vi "Main.vi"() -> ()   [LabVIEW 2019]
doc: "This template is for the Queued Message Handler design pattern.\n\nThe Event Handling Loop generates messages based on user interface actions.\n\nThe Message Handling Loop processes messages generated by the Event Handling Loop, or by other messages. The messages are string values, so new messages can be added easily to the Message Cases case structure in the Message Handling Loop. Each message cluster can also provide an optional value for Message Data, which is a variant that can be converted to whatever message-specific data is required."
uses:
  Firebase.lvclass
  controls/UI Data.ctl
  support/Message Queue/Enqueue Message (Single).vi
  <vilib>/Platform/browser.llb/Open URL in Default Browser (string).vi
  <vilib>/Utility/error.llb/Error Cluster From Error Code.vi
  <vilib>/ErrorRing/Error Ring.xnode
  support/Message Queue/Message Queue.lvlib
  support/User Event - Stop/User Event - Stop.lvlib
panel:
  in  "OPERARIO":string
  in  "Firebase in":refnum<class "Firebase.lvclass">
  out "Firebase out":refnum<class "Firebase.lvclass">
  in  "HUMEDAD ACTUAL":dbl
  in  "TEMPERATURA ACTUAL":dbl
  in  "PH ACTUAL":dbl
  in  "VER BASE DE DATOS":bool
  in  "ACTUALIZAR HUMEDAD":bool
  in  "ACTUALIZAR TEMPERATURA":bool
  in  "ACTUALIZAR PH":bool
  in  "Exit":bool
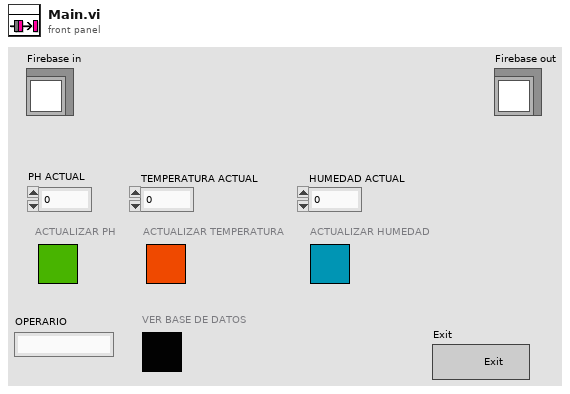
[diagram p1: front panel]
types:
  T1 = typedef "UI Data.ctl" = cluster{"Boolean <Replace Me>":bool, "String <Replace Me>":string, "Numeric <Replace Me>":dbl, "Do Something Ref":refnum<vi>, "Do Something Else Ref":refnum<vi>, "Data Display Ref":refnum<vi>, "Exit Button Ref":refnum<vi>, "OPERARIO":string, "url":string}
  T2 = typedef "Message Queue.lvlib/All Message Queues.ctl" = cluster{"UI":refnum<queue>}
  T3 = cluster{"Fecha":timestamp, "PH":dbl, "Humeda":dbl, "Temperatura":dbl, "Operario":string}
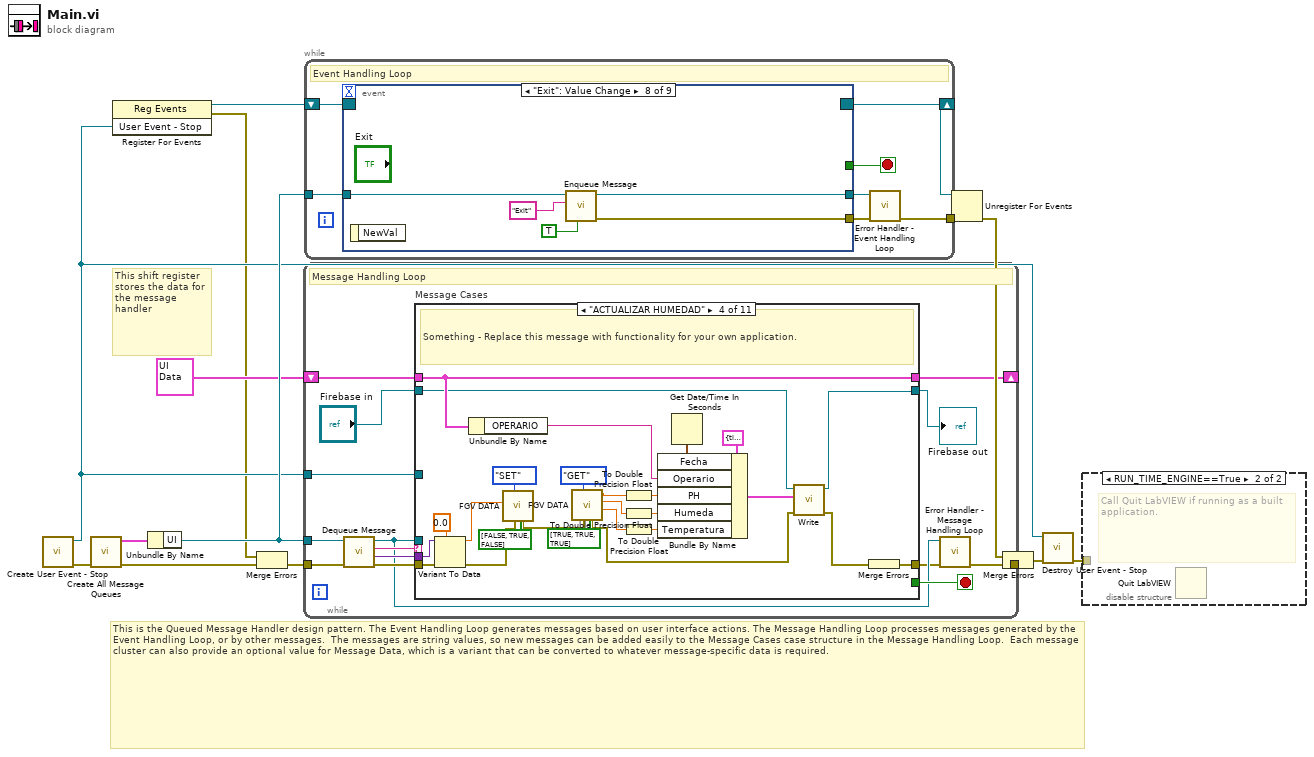
[diagram p0: block diagram]
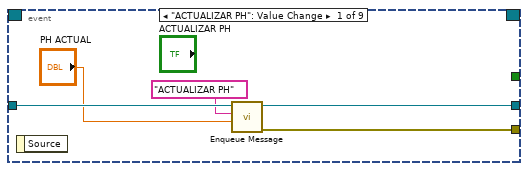
[diagram p3: hidden frame]
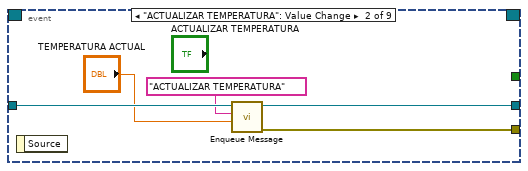
[diagram p4: hidden frame]
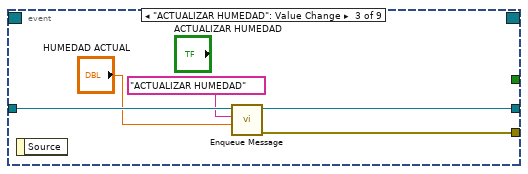
[diagram p5: hidden frame]
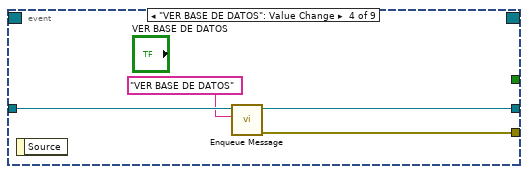
[diagram p6: hidden frame]
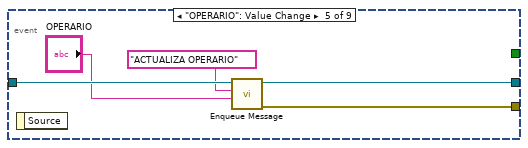
[diagram p7: hidden frame]
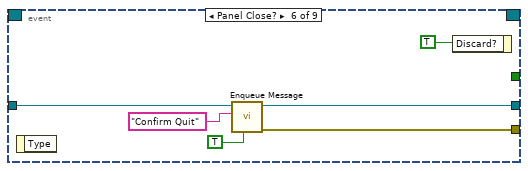
[diagram p8: hidden frame]
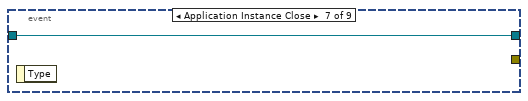
[diagram p9: hidden frame]
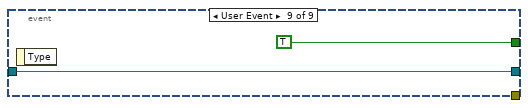
[diagram p10: hidden frame]
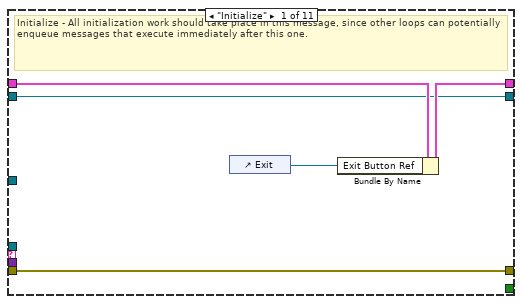
[diagram p11: hidden frame]
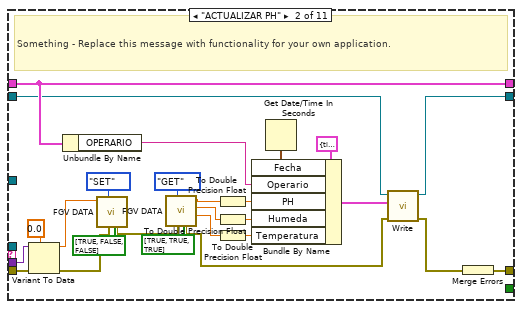
[diagram p12: hidden frame]
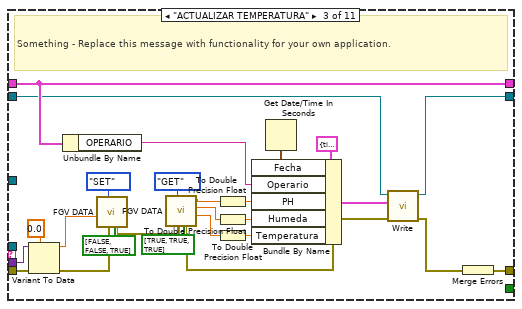
[diagram p13: hidden frame]
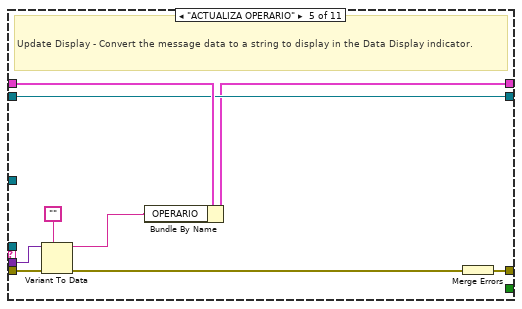
[diagram p14: hidden frame]
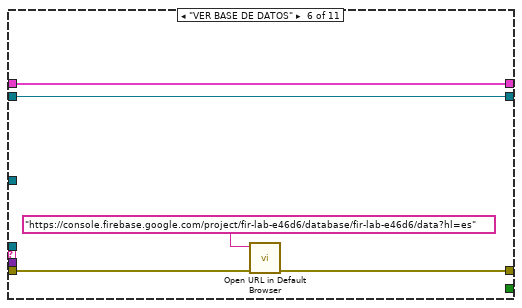
[diagram p15: hidden frame]
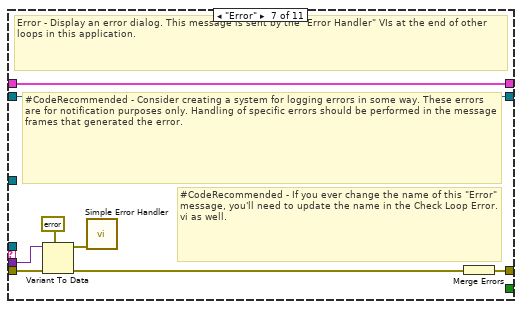
[diagram p16: hidden frame]
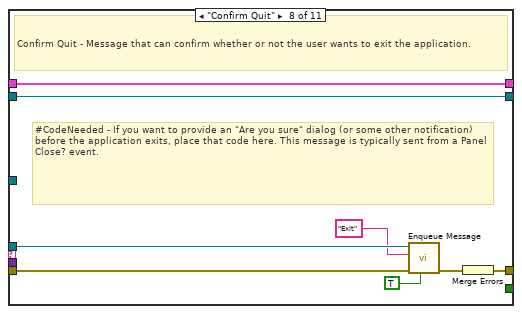
[diagram p17: hidden frame]
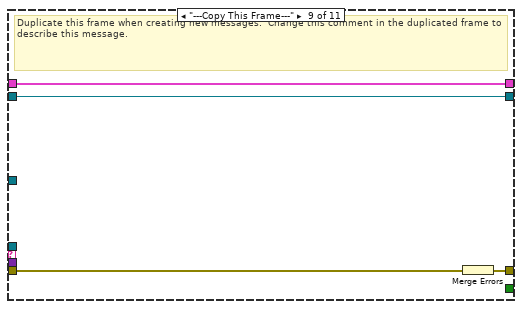
[diagram p18: hidden frame]
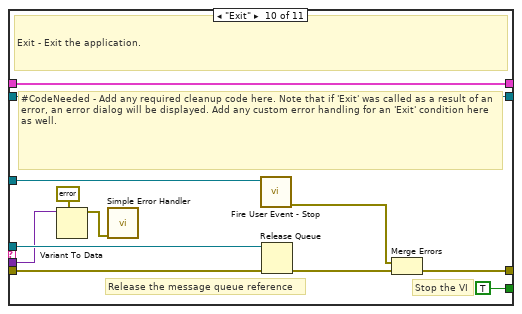
[diagram p19: hidden frame]
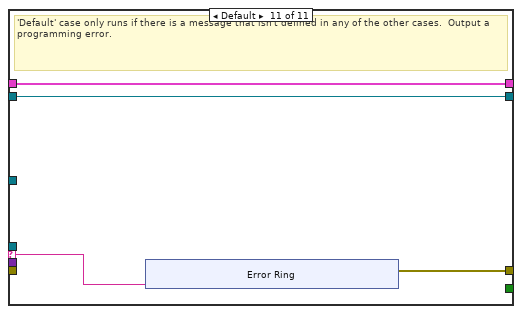
[diagram p20: hidden frame]
diagram:
  # "This is the Queued Message Handler design pattern. The Event Handling Loop generates messages based on user interface actions. The Message Handling Loop processes messages generated by the Event Handling Loop, or by other messages.  The messages are string values, so new messages can be added easily to the Message Cases case structure in the Message Handling Loop.  Each message cluster can also provide an optional value for Message Data, which is a variant that can be converted to whatever message-specific data is required."
  # "This shift register stores the data for the message handler"
  n1 = call "Create User Event - Stop.vi"() -> ("error out"=w11:errorcluster, "User Event - Stop"=w3:refnum<user-event>)  [unwired: 10 in]
  n2 = call "Create All Message Queues.vi"("error in (no error)"=w11) -> ("error out"=w15:errorcluster, "Message Queues out"=w14:T2)  [unwired: 9 in]
  n3 = register-events(w3) -> (reference out=w4:refnum<event-registration>, error out=w1:errorcluster)  [unwired: 2 in]
  n4 = Unbundle By Name(w14) -> ("UI"=w12:refnum<queue>)
  n5 = Merge Errors(w1, w15) -> (w2:errorcluster)
  n6 = while {
    tunnel: w12 -> [w21]
    shift-right: [w28] -> _
    shift-left: T1 {"Boolean <Replace Me>"=FALSE, "String <Replace Me>"="", "Numeric <Replace Me>"=0.0, "Do Something Ref"=refnum, "Do Something Else Ref"=refnum, "Data Display Ref"=refnum, "Exit Button Ref"=refnum, "OPERARIO"="", "url"=""} ("Data Cluster") -> [w29]
    tunnel: w3 -> [w26]
    tunnel: w2 -> [w25]
    tunnel: [w19] -> w13
    stop <- w27 stop-if-true
    # "Message Handling Loop"
    n7 = call "Dequeue Message.vi"("error in (no error)"=w25, "Message Queue"=w21) -> ("error out"=w24:errorcluster, "Message Data"=w22:variant, "Message"=w23:string, "dup Message Queue"=w20:refnum<queue>)  [unwired: 6 in]
    n8 = case "Message Cases" shown="\"ACTUALIZAR HUMEDAD\"" w23 {
      selector: w23 -> [_ _ _ _ _ _ _ _ _ _ w160]
      tunnel: w20 -> [_ _ _ _ _ _ _ w138 _ w158 _]
      tunnel: w24 -> [w34 w59 w85 w111 w119 w123 w134 w142 w146 w151 _]
      tunnel: [w34 w60 w86 w112 w120 w122 w128 w140 w144 w154 w161] -> w18
      tunnel: w29 -> [w33 w43 w71 w96 w121 w126 w133 w141 w145 w157 w162]
      tunnel: [w32 w43 w71 w96 w114 w126 w133 w141 w145 w157 w162] -> w28
      tunnel: [_ _ _ _ _ _ _ _ _ TRUE _] -> w27
      tunnel: w22 -> [_ w38 w66 w92 w118 _ w132 _ _ w148 _]
      tunnel: w26 -> [_ _ _ _ _ _ _ _ _ w153 _]
      tunnel: [w30 w40 w68 w90 w115 w125 w127 w135 w143 w147 w159] -> w17
      tunnel: "Firebase in" -> [w30 w41 w69 w94 w115 w125 w127 w135 w143 w147 w159]
      frame "Initialize" {
        # "Initialize - All initialization work should take place in this message, since other loops can potentially enqueue messages that execute immediately after this one."
        n9 = control-ref of="Exit"() -> (w31:refnum<vi>)
        n10 = Bundle By Name(cluster=w33, "Exit Button Ref"=w31) -> (w32:T1)
      }
      frame "ACTUALIZAR PH" {
        # "Something - Replace this message with functionality for your own application."
        n11 = Variant To Data(error in=w59, type=0.0, Variant=w38) -> (data=w56:dbl, error out=w37:errorcluster)
        n12 = Unbundle By Name(w43) -> ("OPERARIO"=w42:string)
        n13 = call "FGV DATA.vi"("error in (no error)"=w37, "Enum"=enum16{"SET", "GET"}."SET", "SET??"=bool[] [TRUE, FALSE, FALSE], "PH IN"=w56) -> ("error out"=w36:errorcluster)  [unwired: 4 in, 3 out]
        n14 = call "FGV DATA.vi"("error in (no error)"=w36, "Enum"=enum16{"SET", "GET"}."GET", "SET??"=bool[] [TRUE, TRUE, TRUE]) -> ("TEMPERATURA OUT"=w47:dbl, "HUMEDAD OUT"=w48:dbl, "PH OUT"=w49:dbl, "error out"=w35:errorcluster)  [unwired: 5 in]
        n15 = To Double Precision Float(number=w49) -> (double precision float=w50:dbl)
        n16 = To Double Precision Float(number=w48) -> (double precision float=w51:dbl)
        n17 = To Double Precision Float(number=w47) -> (double precision float=w52:dbl)
        n18 = Get Date/Time In Seconds() -> (seconds since 1Jan1904=w44:timestamp)
        n19 = Bundle By Name(cluster=T3 {"Fecha"=timestamp(0 s since 1904-01-01), "PH"=0.0, "Humeda"=0.0, "Temperatura"=0.0, "Operario"=""} ("dato"), "Fecha"=w44, "Operario"=w42, "PH"=w50, "Humeda"=w51, "Temperatura"=w52) -> (w45:T3)
        n20 = call "Write.vi"("error in (no error)"=w35, "dato"=w45, "Firebase in"=w41) -> ("error out"=w39:errorcluster, "Firebase out"=w40:refnum<class "Firebase.lvclass">)  [unwired: 6 in, 1 out]
        n21 = Merge Errors(w39) -> (w60:errorcluster)
      }
      frame "ACTUALIZAR TEMPERATURA" {
        # "Something - Replace this message with functionality for your own application."
        n22 = Variant To Data(error in=w85, type=0.0, Variant=w66) -> (data=w65:dbl, error out=w63:errorcluster)
        n23 = Unbundle By Name(w71) -> ("OPERARIO"=w70:string)
        n24 = call "FGV DATA.vi"("error in (no error)"=w63, "Enum"=enum16{"SET", "GET"}."SET", "SET??"=bool[] [FALSE, FALSE, TRUE], "TEMPERATURA IN"=w65) -> ("error out"=w62:errorcluster)  [unwired: 4 in, 3 out]
        n25 = call "FGV DATA.vi"("error in (no error)"=w62, "Enum"=enum16{"SET", "GET"}."GET", "SET??"=bool[] [TRUE, TRUE, TRUE]) -> ("TEMPERATURA OUT"=w75:dbl, "HUMEDAD OUT"=w76:dbl, "PH OUT"=w77:dbl, "error out"=w61:errorcluster)  [unwired: 5 in]
        n26 = To Double Precision Float(number=w77) -> (double precision float=w78:dbl)
        n27 = To Double Precision Float(number=w76) -> (double precision float=w79:dbl)
        n28 = To Double Precision Float(number=w75) -> (double precision float=w80:dbl)
        n29 = Get Date/Time In Seconds() -> (seconds since 1Jan1904=w72:timestamp)
        n30 = Bundle By Name(cluster=T3 {"Fecha"=timestamp(0 s since 1904-01-01), "PH"=0.0, "Humeda"=0.0, "Temperatura"=0.0, "Operario"=""} ("dato"), "Fecha"=w72, "Operario"=w70, "PH"=w78, "Humeda"=w79, "Temperatura"=w80) -> (w73:T3)
        n31 = call "Write.vi"("error in (no error)"=w61, "dato"=w73, "Firebase in"=w69) -> ("error out"=w67:errorcluster, "Firebase out"=w68:refnum<class "Firebase.lvclass">)  [unwired: 6 in, 1 out]
        n32 = Merge Errors(w67) -> (w86:errorcluster)
      }
      frame "ACTUALIZAR HUMEDAD" {
        # "Something - Replace this message with functionality for your own application."
        n33 = Variant To Data(error in=w111, type=0.0, Variant=w92) -> (data=w91:dbl, error out=w89:errorcluster)
        n34 = Unbundle By Name(w96) -> ("OPERARIO"=w95:string)
        n35 = call "FGV DATA.vi"("error in (no error)"=w89, "Enum"=enum16{"SET", "GET"}."SET", "SET??"=bool[] [FALSE, TRUE, FALSE], "HUMEDAD IN"=w91) -> ("error out"=w88:errorcluster)  [unwired: 4 in, 3 out]
        n36 = call "FGV DATA.vi"("error in (no error)"=w88, "Enum"=enum16{"SET", "GET"}."GET", "SET??"=bool[] [TRUE, TRUE, TRUE]) -> ("TEMPERATURA OUT"=w100:dbl, "HUMEDAD OUT"=w101:dbl, "PH OUT"=w102:dbl, "error out"=w87:errorcluster)  [unwired: 5 in]
        n37 = To Double Precision Float(number=w102) -> (double precision float=w103:dbl)
        n38 = To Double Precision Float(number=w101) -> (double precision float=w104:dbl)
        n39 = To Double Precision Float(number=w100) -> (double precision float=w105:dbl)
        n40 = Get Date/Time In Seconds() -> (seconds since 1Jan1904=w97:timestamp)
        n41 = Bundle By Name(cluster=T3 {"Fecha"=timestamp(0 s since 1904-01-01), "PH"=0.0, "Humeda"=0.0, "Temperatura"=0.0, "Operario"=""} ("dato"), "Fecha"=w97, "Operario"=w95, "PH"=w103, "Humeda"=w104, "Temperatura"=w105) -> (w98:T3)
        n42 = call "Write.vi"("error in (no error)"=w87, "dato"=w98, "Firebase in"=w94) -> ("error out"=w93:errorcluster, "Firebase out"=w90:refnum<class "Firebase.lvclass">)  [unwired: 6 in, 1 out]
        n43 = Merge Errors(w93) -> (w112:errorcluster)
      }
      frame "ACTUALIZA OPERARIO" {
        # "Update Display - Convert the message data to a string to display in the Data Display indicator."
        n44 = Variant To Data(error in=w119, type="", Variant=w118) -> (data=w113:string, error out=w116:errorcluster)
        n45 = Bundle By Name(cluster=w121, "OPERARIO"=w113) -> (w114:T1)
        n46 = Merge Errors(w116) -> (w120:errorcluster)
      }
      frame "VER BASE DE DATOS" {
        n47 = call-poly <vilib>:"Open URL in Default Browser.vi"("error in (no error)"=w123, "URL"="https://console.firebase.google.com/project/fir-lab-e46d6/database/fir-lab-e46d6/data?hl=es") -> ("error out"=w122:errorcluster)  [unwired: 4 in, 1 out]
      }
      frame "Error" {
        # "#CodeRecommended - If you ever change the name of this \"Error\" message, you'll need to update the name in the Check Loop Error.vi as well."
        # "#CodeRecommended - Consider creating a system for logging errors in some way. These errors are for notification purposes only. Handling of specific errors should be performed in the message frames that generated the error."
        # "Error - Display an error dialog. This message is sent by the \"Error Handler\" VIs at the end of other loops in this application."
        n48 = Variant To Data(error in=w134, type=errorcluster {"status"=FALSE, "code"=0, "source"=""} ("error constant"), Variant=w132) -> (data=w130:errorcluster, error out=w129:errorcluster)
        n49 = call <vilib>:"Simple Error Handler.vi"("error in (no error)"=w130) -> ()  [unwired: 4 in, 5 out]
        n50 = Merge Errors(w129) -> (w128:errorcluster)
      }
      frame "Confirm Quit" {
        # "#CodeNeeded - If you want to provide an \"Are you sure\" dialog (or some other notification) before the application exits, place that code here. This message is typically sent from a Panel Close? event."
        # "Confirm Quit - Message that can confirm whether or not the user wants to exit the application."
        n51 = call-poly "Enqueue Message.vi"("Priority Message? (F)"=TRUE, "error in (no error)"=w142, "Message"="Exit", "Message Queue"=w138) -> ("error out"=w139:errorcluster)  [unwired: 6 in, 1 out]
        n52 = Merge Errors(w139) -> (w140:errorcluster)
      }
      frame "---Copy This Frame---" {
        # "Duplicate this frame when creating new messages.  Change this comment in the duplicated frame to describe this message."
        n53 = Merge Errors(w146) -> (w144:errorcluster)
      }
      frame "Exit" {
        # "Stop the VI"
        # "Release the message queue reference"
        # "#CodeNeeded - Add any required cleanup code here. Note that if 'Exit' was called as a result of an error, an error dialog will be displayed. Add any custom error handling for an 'Exit' condition here as well."
        # "Exit - Exit the application."
        n54 = Variant To Data(type=errorcluster {"status"=FALSE, "code"=0, "source"=""} ("error constant"), Variant=w148) -> (data=w149:errorcluster)  [unwired: 1 in, 1 out]
        n55 = call <vilib>:"Simple Error Handler.vi"("error in (no error)"=w149) -> ()  [unwired: 4 in, 5 out]
        n56 = call "Fire User Event - Stop.vi"("User Event - Stop"=w153) -> ("error out"=w152:errorcluster)  [unwired: 10 in]
        n57 = Release Queue(queue=w158, error in (no error)=w151) -> (error out=w155:errorcluster)  [unwired: 1 in, 2 out]
        n58 = Merge Errors(w152, w155) -> (w154:errorcluster)
      }
      frame Default {
        # "'Default' case only runs if there is a message that isn't defined in any of the other cases.  Output a programming error."
        n59 = xnode "Error Ring"("parameter 0"=w160) -> ("error out"=w161:errorcluster)
      }
    }
    "Firebase out" <- w17
    n60 = call "Error Handler - Message Handling Loop.vi"("error in (no error)"=w18, "Message Queue"=w20) -> ("dup error in"=w19:errorcluster)  [unwired: 8 in, 1 out]
  }
  n61 = while {
    tunnel: w12 -> [w176]
    shift-right: [w174] -> w8
    shift-left: w4 -> [w175]
    tunnel: [w170] -> w5
    stop <- w172 stop-if-true
    # "Event Handling Loop"
    n62 = event shown="[7] \"Exit\": Value Change" {
      selector: w175 -> [_ _ _ _ _ _ _ _ _]
      dyn-events: [_ _ _ _ _ _ _ _ _] -> w174
      timeout: _ -> [_ _ _ _ _ _ _ _ _]
      tunnel: [_ _ _ _ _ _ _ _ TRUE ("Discard?")] -> w172
      tunnel: w176 -> [w181 w186 w191 w195 w200 w205 w207 w212 w214]
      tunnel: [w178 w183 w188 w192 w197 w204 _ w211 _] -> w173
      tunnel: [w180 w185 w190 w194 w199 w203 w207 w210 w214] -> w171
      event "ACTUALIZAR PH": Value Change {
        n63 = event-data() -> ()  [unwired: 1 in, 1 out]
        n64 = call-poly "Enqueue Message.vi"("Message Data"="PH ACTUAL", "Message"="ACTUALIZAR PH", "Message Queue"=w181) -> ("error out"=w178:errorcluster, "dup Message Queue"=w180:refnum<queue>)  [unwired: 7 in]
      }
      event "ACTUALIZAR TEMPERATURA": Value Change {
        n65 = event-data() -> ()  [unwired: 1 in, 1 out]
        n66 = call-poly "Enqueue Message.vi"("Message Data"="TEMPERATURA ACTUAL", "Message"="ACTUALIZAR TEMPERATURA", "Message Queue"=w186) -> ("error out"=w183:errorcluster, "dup Message Queue"=w185:refnum<queue>)  [unwired: 7 in]
      }
      event "ACTUALIZAR HUMEDAD": Value Change {
        n67 = event-data() -> ()  [unwired: 1 in, 1 out]
        n68 = call-poly "Enqueue Message.vi"("Message Data"="HUMEDAD ACTUAL", "Message"="ACTUALIZAR HUMEDAD", "Message Queue"=w191) -> ("error out"=w188:errorcluster, "dup Message Queue"=w190:refnum<queue>)  [unwired: 7 in]
      }
      event "VER BASE DE DATOS": Value Change {
        n69 = event-data() -> ()  [unwired: 1 in, 1 out]
        n70 = call-poly "Enqueue Message.vi"("Message"="VER BASE DE DATOS", "Message Queue"=w195) -> ("error out"=w192:errorcluster, "dup Message Queue"=w194:refnum<queue>)  [unwired: 8 in]
      }
      event "OPERARIO": Value Change {
        n71 = event-data() -> ()  [unwired: 1 in, 1 out]
        n72 = call-poly "Enqueue Message.vi"("Message Data"="OPERARIO", "Message"="ACTUALIZA OPERARIO", "Message Queue"=w200) -> ("error out"=w197:errorcluster, "dup Message Queue"=w199:refnum<queue>)  [unwired: 7 in]
      }
      event Panel Close? {
        n73 = event-data() -> ()  [unwired: 1 in, 1 out]
        n74 = call-poly "Enqueue Message.vi"("Priority Message? (F)"=TRUE, "Message"="Confirm Quit", "Message Queue"=w205) -> ("error out"=w204:errorcluster, "dup Message Queue"=w203:refnum<queue>)  [unwired: 7 in]
        n75 = event-data("Discard?"=TRUE) -> ()  [unwired: 1 in, 1 out]
      }
      event Application Instance Close {
        n76 = event-data() -> ()  [unwired: 1 in, 1 out]
      }
      event "Exit": Value Change {
        n77 = event-data() -> ()  [unwired: 1 in, 1 out]
        n78 = call-poly "Enqueue Message.vi"("Priority Message? (F)"=TRUE, "Message"="Exit", "Message Queue"=w212) -> ("error out"=w211:errorcluster, "dup Message Queue"=w210:refnum<queue>)  [unwired: 7 in]
      }
      event User Event {
        n79 = event-data() -> ()  [unwired: 1 in, 1 out]
      }
    }
    n80 = call "Error Handler - Event Handling Loop.vi"("error in (no error)"=w173, "Message Queue"=w171) -> ("dup error in"=w170:errorcluster)  [unwired: 8 in, 1 out]
  }
  n81 = Unregister For Events(event registration refnum=w8, error in=w5) -> (error out=w9:errorcluster)
  n82 = Merge Errors(w9, w13) -> (w10:errorcluster)
  n83 = call "Destroy User Event - Stop.vi"("error in (no error)"=w10, "User Event - Stop"=w3) -> ("error out"=w6:errorcluster)  [unwired: 9 in]
  n84 = disable-structure shown="RUN_TIME_ENGINE==True" {
    disable-tunnel: w6 -> [_ _]
    frame condition #0 (active) {
    }
    frame condition #1 {
      # "Call Quit LabVIEW if running as a built application."
      n85 = Quit LabVIEW() -> ()  [unwired: 1 in]
    }
  }
